vi "Generate City Plan Cards.vi"(11 "Path":path) -> (3 "City Plan Cards":variant[](array[variant]))   [LabVIEW 2019]
doc: "Generates an array of all rule cards. Each card is stored as a Variant key-value pairs for the Set (1,2,3), Base (T/F), and Image.\n\nBase=True indicates the card is part of the base game\nBase=False indicates the card is part of the advnced game"
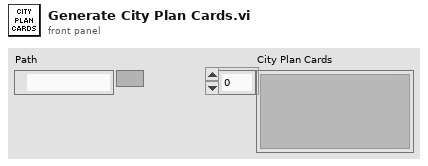
[diagram p1: front panel]
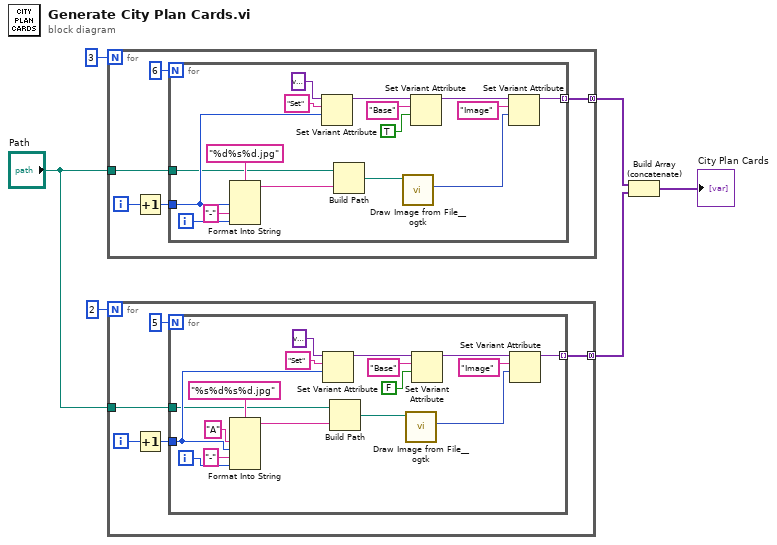
[diagram p0: block diagram]
diagram:
  n1 = for {
    N: 3 -> [_]
    tunnel: "Path" -> [w8]
    tunnel: [w7] -> w3 mode=concatenating
    i -> [w9]
    n2 = Increment(x=w9) -> (x+1=w10:i32)
    n3 = for {
      N: 6 -> [_]
      tunnel: w10 -> [w17]
      tunnel: w8 -> [w16]
      tunnel: [w12] -> w7 mode=indexing
      i -> [w26]
      n4 = Format Into String(format string="%d%s%d.jpg", w17, "-", w26) -> (resulting string=w15:string)  [unwired: 2 in, 1 out]
      n5 = Set Variant Attribute(Variant=variant, name="Set", value=w17) -> (Variant out=w21:variant)  [unwired: 1 in, 2 out]
      n6 = Build Path(base path=w16, name or relative path=w15) -> (appended path=w14:path)
      n7 = call <userlib>:"Draw Image from File__ogtk.vi"("path to image file"=w14) -> ("new picture"=w13:picture)  [unwired: 7 in, 3 out]
      n8 = Set Variant Attribute(Variant=w21, name="Base", value=TRUE) -> (Variant out=w19:variant)  [unwired: 1 in, 2 out]
      n9 = Set Variant Attribute(Variant=w19, name="Image", value=w13) -> (Variant out=w12:variant)  [unwired: 1 in, 2 out]
    }
  }
  n10 = for {
    N: 2 -> [_]
    tunnel: "Path" -> [w29]
    tunnel: [w28] -> w2 mode=concatenating
    i -> [w30]
    n11 = Increment(x=w30) -> (x+1=w31:i32)
    n12 = for {
      N: 5 -> [_]
      tunnel: w31 -> [w38]
      tunnel: w29 -> [w37]
      tunnel: [w33] -> w28 mode=indexing
      i -> [w48]
      n13 = Format Into String(format string="%s%d%s%d.jpg", "A", w38, "-", w48) -> (resulting string=w36:string)  [unwired: 2 in, 1 out]
      n14 = Set Variant Attribute(Variant=variant, name="Set", value=w38) -> (Variant out=w42:variant)  [unwired: 1 in, 2 out]
      n15 = Build Path(base path=w37, name or relative path=w36) -> (appended path=w35:path)
      n16 = call <userlib>:"Draw Image from File__ogtk.vi"("path to image file"=w35) -> ("new picture"=w34:picture)  [unwired: 7 in, 3 out]
      n17 = Set Variant Attribute(Variant=w42, name="Base", value=FALSE) -> (Variant out=w40:variant)  [unwired: 1 in, 2 out]
      n18 = Set Variant Attribute(Variant=w40, name="Image", value=w34) -> (Variant out=w33:variant)  [unwired: 1 in, 2 out]
    }
  }
  n19 = Build Array (concatenate)(w3, w2) -> (→"City Plan Cards":variant[])
